vi "MN_transfer_Z.vi"(4 "x":dbl format="%#_13g") -> (1 "y":dbl)   [LabVIEW 2015]
panel:
  out "x*y 2":dbl[](array[numeric])
  out "Error (mm)":dbl[][](graph)
  out "x*y":dbl[](array[numeric])
  out "array w/ subset deleted":dbl[](array[numeric])
  in  "Nn":dbl[](array[numeric])=[0.0, 9.73217504156629e-05, -0.000306902252647143, 0.000361035276367089, -0.000188468692628135, 3.70139184925173e-05, 8.58351586463287e-18] format="%#_13g"
  in  "Nd":dbl[](array[numeric])=[1.0, -4.44700230387151, 8.24839085487662, -8.14427397698459, 4.49788979210274, -1.31169151684275, 0.15722695108496] format="%#_13g"
  out "yk chain":dbl[](array[numeric])
  out "xk chain":dbl[](array[numeric])
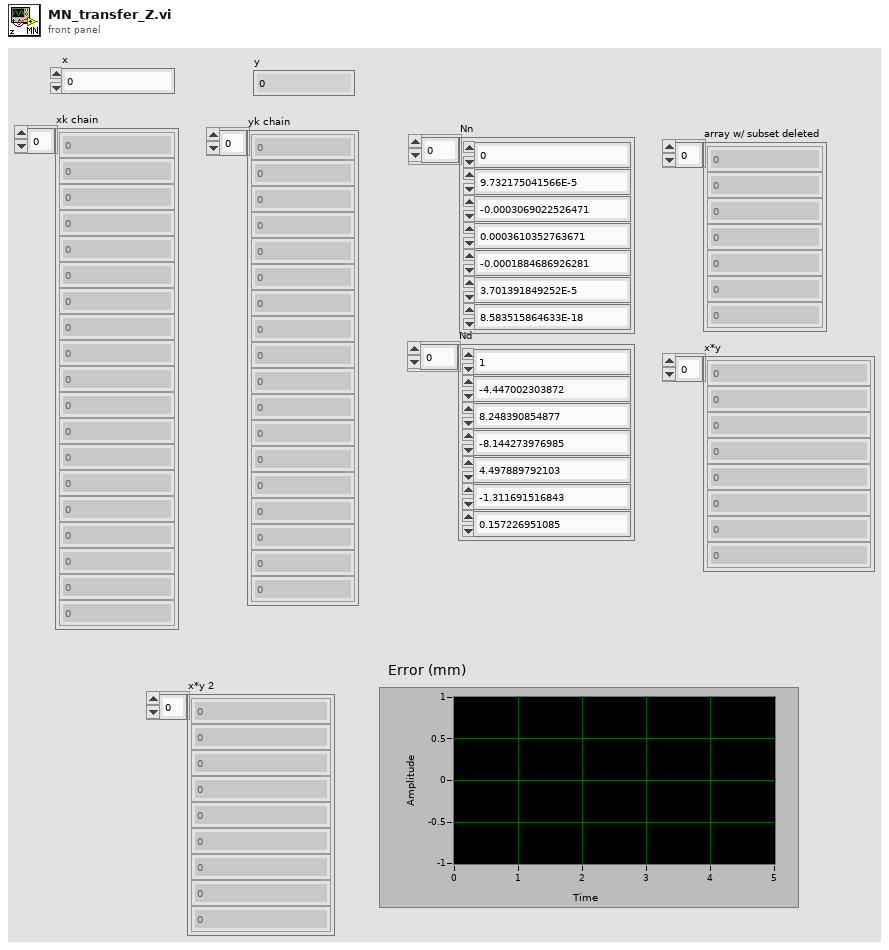
[diagram p1: front panel]
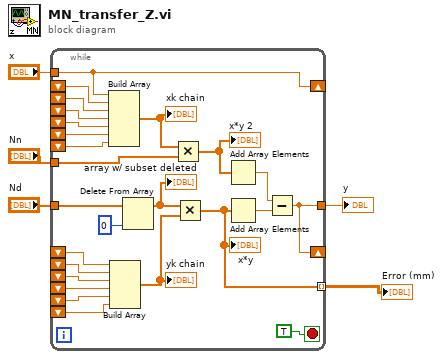
[diagram p0: block diagram]
diagram:
  n1 = while {
    tunnel: [w23] -> w2
    tunnel: "x" -> [w25]
    tunnel: "Nd" -> [w19]
    tunnel: "Nn" -> [w20]
    shift-right: [w25] -> _
    shift-left: _ -> [w24]
    shift-right: [w23] -> _
    shift-left: _ -> [w18]
    shift-left: _ -> [w16]
    shift-left: _ -> [w15]
    shift-left: _ -> [w14]
    shift-left: _ -> [w13]
    shift-left: _ -> [w12]
    shift-left: _ -> [w11]
    tunnel: [w10] -> w3 mode=indexing
    shift-left: _ -> [w9]
    shift-left: _ -> [w8]
    shift-left: _ -> [w6]
    shift-left: _ -> [w7]
    stop <- TRUE stop-if-true
    n2 = Build Array(w25, w24, w13, w12, w11, w9, w6) -> (w21:dbl[])
    "xk chain" <- w21
    n3 = Build Array(w18, w16, w15, w14, w8, w7) -> (w17:dbl[])
    "yk chain" <- w17
    n4 = Delete From Array(array=w19, index=0) -> (array with subset deleted=w28:dbl[])  [unwired: 1 in, 1 out]
    "array w/ subset deleted" <- w28
    n5 = Multiply(x=w21, y=w20) -> (x*y=w30:dbl[])
    "x*y 2" <- w30
    n6 = Multiply(x=w28, y=w17) -> (x*y=w10:dbl[])
    "x*y" <- w10
    n7 = Add Array Elements(numeric array=w30) -> (sum=w27:dbl)
    n8 = Add Array Elements(numeric array=w10) -> (sum=w26:dbl)
    n9 = Subtract(x=w27, y=w26) -> (x-y=w23:dbl)
  }
  "y" <- w2
  "Error (mm)" <- w3
